vi "MotorControl.vi"() -> ()   [LabVIEW 2018]
panel:
  in  "stop":bool
  in  "Motor control":enum32{"Movement", "Setup", "Error"}(tab)
  in  "Single motion":bool=TRUE
  out "Step number":i32=1
  out "Motor Relative":dbl[](array[numeric])=[-100.0, -1.0, -1.0, -1.0]
  in  "Speed (mm/s)":dbl[](array[numeric])=[5.0, 5.0, 5.0, 10.0] format="%#_13g"
  in  "Distance  (mm)":dbl[](array[numeric])=[0.0, -100.0, 0.0, 0.0] format="%#_13g"
  in  "Send All":bool
  in  "Stop motion":bool
  out "Moving":bool
  out "Acquiring":bool
  in  "Go to zero":bool
  out "Motor Status":bool
  out "Number of steps":i32=1
  out "Time between steps":dbl format="%#_13g"
  out "run number":i32=37
  in  "Reset motor":bool
  in  "Inc run #":bool
  in  "Send":bool[](array[boolean])=[FALSE, FALSE, FALSE, FALSE]
  in  "Motor zero":dbl[](array[numeric])=[100.0, 1.0, 1.0, 1.0] format="%#_13g"
  out "Motor absolute":dbl[](array[numeric])
  in  "Motor Port":string="COM12 19200"
  in  "Time between steps ctrl":dbl=5.0 caption="Time Target (s)"
  in  "# steps ctrl":i32=3
  in  "Conversion (steps/mm)":dbl[](array[numeric])=[31496.063, 31496.063, 31496.063, 12500.0] format="%#_13g"
  in  "Reset distance after run":bool
  in  "auto inc run #":bool
  in  "Zero":bool[](array[boolean])=[FALSE, FALSE, FALSE, FALSE]
  out "error out":errorcluster={"status"=TRUE, "code"=-2147221164, "source"="Class not registered\r\n in MotorControl - Copy.vi"}
  out "Library Version":string
  out "Connect To:":string
  in  "Galil.IGalil":refnum<k7>
  # "spend time updating output cluster?"
  # "Motor A"
  # "Motor B"
  # "Motor C"
  # "Motor D"
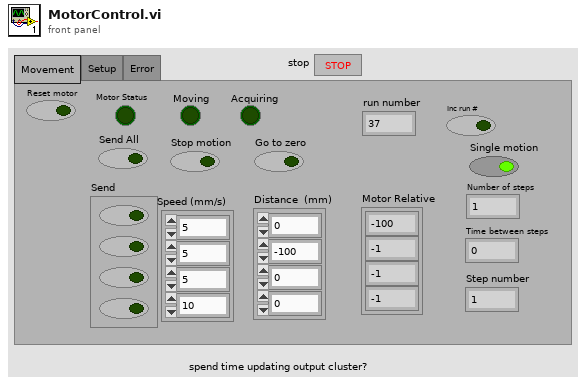
[diagram p1: front panel]
types:
  T1 = enum16{"open", "open or create", "create or replace", "create", "open (read-only)"}
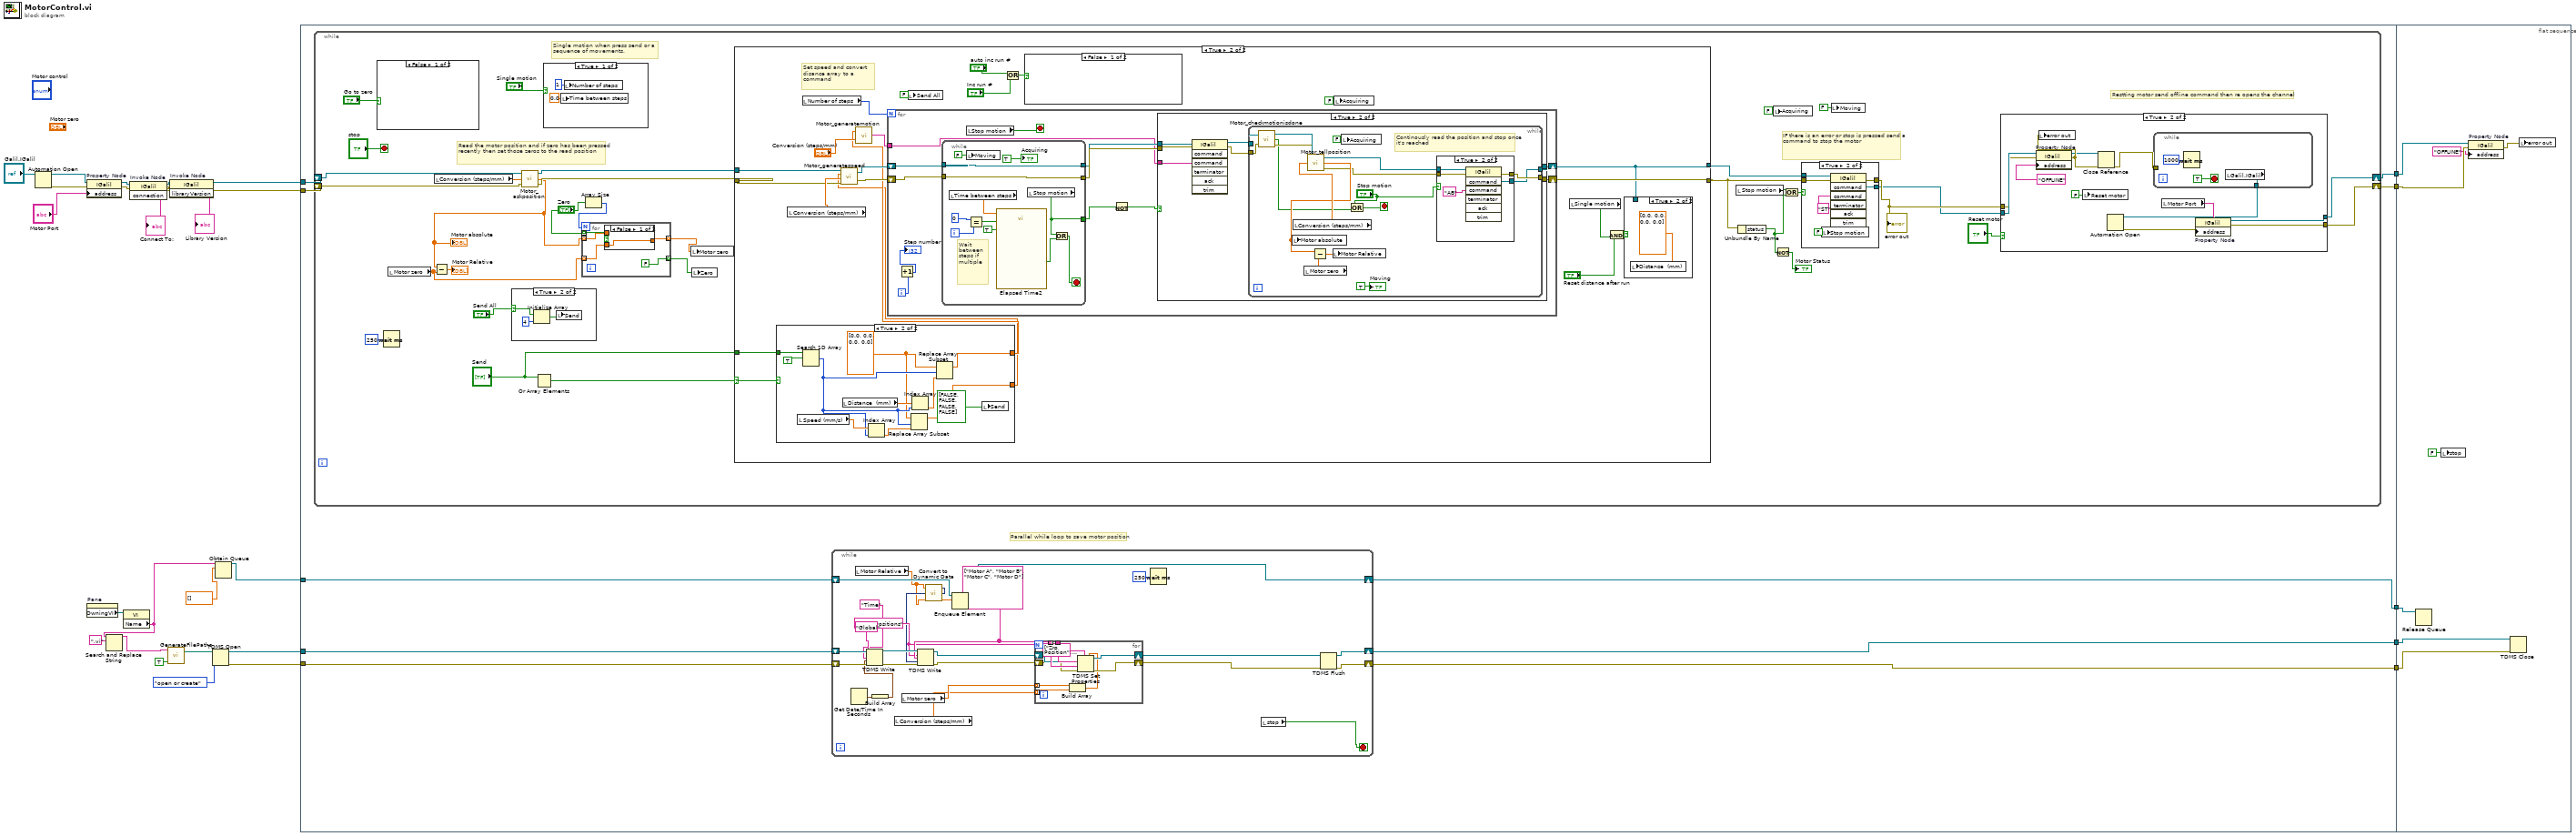
[diagram p0: block diagram]
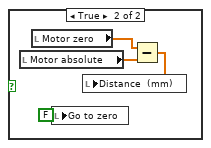
[diagram p5: hidden frame]
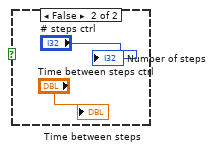
[diagram p7: hidden frame]
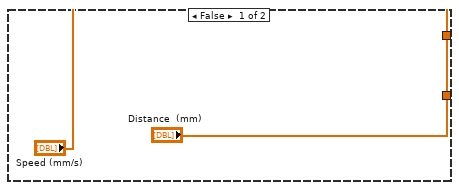
[diagram p9: hidden frame]
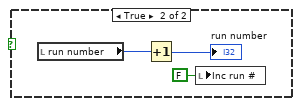
[diagram p10: hidden frame]
diagram:
  n1 = Automation Open(Automation Refnum="Galil.IGalil") -> (Automation Refnum=w22:refnum<k7>, error out=w26:errorcluster)  [unwired: 3 in]
  n2 = property on="Property Node" class="IGalil"(reference=w22, error in=w26, "address"="Motor Port") -> (reference out=w27:refnum<k7>, error out=w25:errorcluster)
  n3 = property on="Pane" class="Pane"() -> ("OwningVI"=w16:refnum<vi>)  [unwired: 2 in, 2 out]
  n4 = property class="VI"(reference=w16) -> ("Name"=w1:string)  [unwired: 1 in, 2 out]
  n5 = Search and Replace String(input string=w1, search string=".vi") -> (result string=w14:string)  [unwired: 6 in, 3 out]
  n6 = invoke on="Invoke Node" class="IGalil" method="connection"(reference=w27, error in=w25) -> (reference out=w21:refnum<k7>, error out=w20:errorcluster, "connection"=→"Connect To:":string)  [unwired: 1 in]
  n7 = call "GenerateFilePaths.vi"("Logfile? (F)"=TRUE ("Logfile?"), "Device Name"=w14) -> ("Path"=w12:path)  [unwired: 3 in]
  n8 = invoke on="Invoke Node" class="IGalil" method="libraryVersion"(reference=w21, error in=w20) -> (reference out=w18:refnum<k7>, error out=w17:errorcluster, "libraryVersion"=→"Library Version":string)  [unwired: 1 in]
  n9 = TDMS Open(10:T1."open or create" ("operation (0:open)"), 11:w12) -> (0:w9:errorcluster, 3:w10:refnum<k34>)  [unwired: 5 in]
  n10 = Obtain Queue(name (unnamed)=w1, element data type=dbl[] []) -> (queue out=w3:refnum<queue>)  [unwired: 3 in, 2 out]
  n11 = flat-sequence {
    tunnel: w18 -> [w38]
    tunnel: w17 -> [w37]
    tunnel: w10 -> [w34]
    tunnel: w9 -> [w33]
    tunnel: [w36] -> w8
    tunnel: [w35] -> w7
    tunnel: [w32] -> w6
    tunnel: [w31] -> w5
    tunnel: w3 -> [w29]
    tunnel: [w30] -> w2
    tunnel: w8 -> [w251]
    tunnel: w7 -> [w250]
    tunnel: w6 -> [w253]
    tunnel: w5 -> [w254]
    tunnel: w2 -> [w247]
    frame #0 {
      # "Parallel while loop to save motor position"
      n12 = while {
        shift-right: [w84] -> w36
        shift-left: w38 -> [w94]
        shift-right: [w83] -> w35
        shift-left: w37 -> [w93]
        stop <- "stop" stop-if-true
        # "Restting motor send offline command then re opens the channel"
        # "IF there is an error or stop is pressed send a command to stop the motor"
        # "Read the motor position and if zero has been pressed recently then set those zeros to the read position"
        # "Single motion when press send or a sequence of movements."
        n13 = case shown="False" "Go to zero" {
          frame False {
          }
          frame True {
            n14 = local read "Motor absolute"() -> (w134:dbl[])
            n15 = local read "Motor zero"() -> (w135:dbl[])
            n16 = local write "Go to zero"(FALSE ("Zero A")) -> ()
            n17 = Subtract(x=w135, y=w134) -> (x-y=w133:dbl[])
            n18 = local write "Distance  (mm)"(w133) -> ()
          }
        }
        n19 = Wait (ms)(milliseconds to wait=u32 250) -> ()  [unwired: 1 out]
        n20 = local read "Motor zero"() -> (w80:dbl[])
        n21 = local read "Conversion (steps/mm)"() -> (w90:dbl[])
        n22 = case shown="True" "Send All" {
          selector: "Send All" -> [_ w106]
          frame False {
          }
          frame True {
            n23 = Initialize Array(w106, 4 ("dimension size")) -> (w105:bool[])
            n24 = local write "Send"(w105) -> ()
          }
        }
        n25 = call "Motor_askposition.vi"("error in (no error)"=w93, "Conversion\n (steps/mm)"=w90, "reference"=w94) -> ("error out"=w91:errorcluster, "position out"=w73:dbl[], "reference out"=w92:refnum<k7>)
        "Motor absolute" <- w73
        n26 = Subtract(x=w73, y=w80) -> (x-y=→"Motor Relative":dbl[])
        n27 = Or Array Elements(Boolean array="Send") -> (logical OR=w77:bool)
        n28 = case shown="True" "Single motion" {
          frame True {
            n29 = local write "Time between steps"(0.0 ("Time between steps")) -> ()
            n30 = local write "Number of steps"(1 ("Number of steps")) -> ()
          }
          frame False {
            "Number of steps" <- "# steps ctrl"
            "Time between steps" <- "Time between steps ctrl"
          }
        }
        n31 = Array Size(array="Zero") -> (size(s)=w74:i32)
        n32 = for {
          N: w74 -> [_]
          tunnel: w73 -> [w112] mode=indexing
          tunnel: [FALSE ("Boolean")] -> w81 mode=indexing
          tunnel: "Zero" -> [w111] mode=indexing
          tunnel: [w110] -> w79 mode=indexing
          tunnel: w80 -> [w109] mode=indexing
          n33 = case shown="False" w111 {
            tunnel: w112 -> [_ w114]
            tunnel: [w113 w114] -> w110
            tunnel: w109 -> [w113 _]
            frame False {
            }
            frame True {
            }
          }
        }
        n34 = local write "Motor zero"(w79) -> ()
        n35 = local write "Zero"(w81) -> ()
        n36 = case shown="True" w77 {
          selector: w77 -> [_ w151]
          tunnel: w92 -> [w150 w164]
          tunnel: w91 -> [w149 w163]
          tunnel: [w150 w165] -> w98
          tunnel: [w149 w171] -> w95
          tunnel: "Send" -> [_ w154]
          frame False {
          }
          frame True {
            # "Set speed and convert disance array to a command"
            n37 = case shown="True" w151 {
              tunnel: w154 -> [_ w181]
              tunnel: ["Distance  (mm)" w180] -> w153
              tunnel: ["Speed (mm/s)" w176] -> w152
              frame False {
              }
              frame True {
                w175 = dbl[] [0.0, 0.0, 0.0, 0.0]
                n38 = local read "Speed (mm/s)"() -> (w178:dbl[])
                n39 = Search 1D Array(1D array=w181, element=TRUE) -> (index of element=w177:i32)  [unwired: 1 in]
                n40 = local read "Distance  (mm)"() -> (w183:dbl[])
                n41 = Index Array(array=w178, index=w177) -> (element=w179:dbl)
                n42 = Replace Array Subset(array=w175, new element=w179, index=w177) -> (w176:dbl[])
                n43 = Index Array(array=w183, index=w177) -> (element=w185:dbl)
                n44 = Replace Array Subset(array=w175, new element=w185, index=w177) -> (w180:dbl[])
                n45 = local write "Send"(bool[] [FALSE, FALSE, FALSE, FALSE]) -> ()
              }
            }
            n46 = local read "Conversion (steps/mm)"() -> (w166:dbl[])
            n47 = local read "Number of steps"() -> (w169:i32)
            n48 = call "Motor_generatespeed.vi"("error in (no error)"=w163, "Conversion\n (steps/mm)"=w166, "Speed (mm/s)"=w152, "reference"=w164) -> ("error out"=w161:errorcluster, "reference out"=w162:refnum<k7>)
            n49 = call "Motor_generatemotion.vi"("Conversion\n (steps/mm)"="Conversion (steps/mm)", "Distance  (mm)"=w153) -> ("Movement String"=w167:string)
            n50 = for {
              N: w169 -> [_]
              tunnel: w167 -> [w190]
              shift-right: [w196] -> w165
              shift-left: w162 -> [w198]
              shift-right: [w195] -> w171
              shift-left: w161 -> [w197]
              i -> [w200]
              stop <- w201 stop-if-true
              n51 = Increment(x=w200) -> (x+1=→"Step number":i32)
              n52 = while {
                tunnel: w198 -> [w245]
                tunnel: [w246] -> w192
                tunnel: w197 -> [w246]
                tunnel: [w245] -> w191
                tunnel: [w235] -> w193
                i -> [w241]
                stop <- w243 stop-if-true
                # "Wait between steps if multiple"
                n53 = local read "Time between steps"() -> (w237:dbl)
                n54 = local write "Moving"(FALSE ("Aquiring")) -> ()
                n55 = Equal?(x=0, y=w241) -> (x = y?=w239:bool)
                n56 = call "Elapsed Time2"("Time Target (s)"=w237, "Reset"=w239, "Auto Reset"=TRUE) -> ("Time has Elapsed"=w244:bool)  [unwired: 9 in, 7 out]
                n57 = local read "Stop motion"() -> (w235:bool)
                n58 = Or(x=w235, y=w244) -> (x .or. y?=w243:bool)
                "Acquiring" <- TRUE
              }
              n59 = local read "Stop motion"() -> (w201:bool)
              n60 = Not(x=w193) -> (.not. x?=w194:bool)
              n61 = case shown="True" w194 {
                tunnel: w191 -> [w203 w208]
                tunnel: w192 -> [w202 w205]
                tunnel: [w203 w210] -> w196
                tunnel: [w202 w209] -> w195
                tunnel: w190 -> [_ w204]
                frame False {
                }
                frame True {
                  n62 = invoke class="IGalil" method="command"(reference=w208, error in=w205, "command"=w204) -> (reference out=w207:refnum<k7>, error out=w206:errorcluster)  [unwired: 4 in, 5 out]
                  n63 = while {
                    tunnel: w207 -> [w220]
                    tunnel: [w213] -> w210
                    tunnel: [w214] -> w209
                    tunnel: w206 -> [w211]
                    stop <- w226 stop-if-true
                    # "Continously read the position and stop once it's reached"
                    n64 = call "Motor_checkmotionisdone.vi"("reference"=w220, "error in (no error)"=w211) -> ("reference out"=w219:refnum<k7>, "Motion is done"=w217:bool, "error out"=w218:errorcluster)
                    n65 = local read "Conversion (steps/mm)"() -> (w222:dbl[])
                    n66 = local read "Motor zero"() -> (w225:dbl[])
                    n67 = call "Motor_tellposition.vi"("error in (no error)"=w218, "Conversion\n (steps/mm)"=w222, "reference"=w219) -> ("error out"=w215:errorcluster, "Position out"=w221:dbl[], "reference out"=w216:refnum<k7>)
                    n68 = local write "Motor absolute"(w221) -> ()
                    n69 = Subtract(x=w221, y=w225) -> (x-y=w224:dbl[])
                    n70 = local write "Motor Relative"(w224) -> ()
                    n71 = local write "Acquiring"(FALSE ("Aquiring")) -> ()
                    n72 = Or(x="Stop motion", y=w217) -> (x .or. y?=w226:bool)
                    n73 = case shown="True" "Stop motion" {
                      tunnel: w216 -> [w229 w233]
                      tunnel: w215 -> [w228 w232]
                      tunnel: [w229 w231] -> w213
                      tunnel: [w228 w230] -> w214
                      frame False {
                      }
                      frame True {
                        n74 = invoke class="IGalil" method="command"(reference=w233, error in=w232, "command"="AB") -> (reference out=w231:refnum<k7>, error out=w230:errorcluster)  [unwired: 4 in, 5 out]
                      }
                    }
                    "Moving" <- TRUE
                  }
                }
              }
            }
            n75 = local write "Send All"(FALSE ("Send")) -> ()
            n76 = Or(x="auto inc run #", y="Inc run #") -> (x .or. y?=w157:bool)
            n77 = case shown="False" w157 {
              frame False {
              }
              frame True {
                n78 = local read "run number"() -> (w187:i32)
                n79 = Increment(x=w187) -> (x+1=→"run number":i32)
                n80 = local write "Inc run #"(FALSE ("Inc run #")) -> ()
              }
            }
            n81 = local write "Acquiring"(FALSE ("Aquiring")) -> ()
            n82 = local read "Single motion"() -> (w159:bool)
            n83 = And(x="Reset distance after run", y=w159) -> (x .and. y?=w160:bool)
            n84 = case shown="True" w160 {
              tunnel: w165 -> [_ _]
              frame False {
              }
              frame True {
                n85 = local write "Distance  (mm)"(dbl[] [0.0, 0.0, 0.0, 0.0] ("Distance  (mm)")) -> ()
              }
            }
          }
        }
        n86 = local read "Stop motion"() -> (w96:bool)
        n87 = Unbundle By Name(w95) -> ("status"=w88:bool)
        n88 = local write "Acquiring"(FALSE ("Aquiring")) -> ()
        n89 = Not(x=w88) -> (.not. x?=→"Motor Status":bool)
        n90 = Or(x=w96, y=w88) -> (x .or. y?=w97:bool)
        n91 = case shown="True" w97 {
          tunnel: w98 -> [w138 w143]
          tunnel: w95 -> [w137 w142]
          tunnel: [w138 w141] -> w85
          tunnel: [w137 w140] -> w86
          frame False {
          }
          frame True {
            n92 = local write "Stop motion"(FALSE ("Stop motion")) -> ()
            n93 = invoke class="IGalil" method="command"(reference=w143, error in=w142, "command"="ST") -> (reference out=w141:refnum<k7>, error out=w140:errorcluster)  [unwired: 4 in, 5 out]
          }
        }
        "error out" <- w86
        n94 = local write "Moving"(FALSE ("Waiting")) -> ()
        n95 = case shown="True" "Reset motor" {
          tunnel: w85 -> [w115 w118]
          tunnel: w86 -> [w116 w117]
          tunnel: [w115 w128] -> w84
          tunnel: [w116 w129] -> w83
          frame False {
          }
          frame True {
            n96 = property on="Property Node" class="IGalil"(reference=w118, error in=w117, "address"="OFFLINE") -> (reference out=w121:refnum<k7>, error out=w122:errorcluster)
            n97 = local write "error out"(w122) -> ()
            n98 = local write "Reset motor"(FALSE ("Reset motor")) -> ()
            n99 = Close Reference(reference=w121, error in (no error)=w122) -> (error out=w119:errorcluster)
            n100 = while {
              tunnel: [w130] -> w126
              tunnel: w119 -> [_]
              stop <- TRUE stop-if-true
              n101 = Wait (ms)(milliseconds to wait=u32 1000) -> ()  [unwired: 1 out]
              n102 = local read "Galil.IGalil"() -> (w130:refnum<k7>)
            }
            n103 = Automation Open(Automation Refnum=w126) -> (Automation Refnum=w125:refnum<k7>, error out=w124:errorcluster)  [unwired: 3 in]
            n104 = local read "Motor Port"() -> (w127:string)
            n105 = property on="Property Node" class="IGalil"(reference=w125, error in=w124, "address"=w127) -> (reference out=w128:refnum<k7>, error out=w129:errorcluster)
          }
        }
      }
      n106 = while {
        shift-right: [w47] -> w32
        shift-left: w34 -> [w62]
        shift-right: [w48] -> w31
        shift-left: w33 -> [w61]
        shift-right: [w40] -> w30
        shift-left: w29 -> [w41]
        stop <- w46 stop-if-true
        w54 = string[] ["Motor A", "Motor B", "Motor C", "Motor D"]
        w53 = "Motor Positions" ("group name in (Untitled)")
        n107 = Get Date/Time In Seconds() -> (seconds since 1Jan1904=w58:timestamp)
        n108 = local read "Motor Relative"() -> (w39:dbl[])
        n109 = Build Array(w58) -> (w57:timestamp[])
        n110 = TDMS Write(0:w62, 5:"Global" ("group name in (Untitled)"), 7:"Time" ("group name in (Untitled)"), 9:w57, 11:w61) -> (4:w56:refnum<k34>, 15:w55:errorcluster)  [unwired: 1 in, 2 out]
        n111 = local read "Conversion (steps/mm)"() -> (w42:dbl[])
        n112 = local read "Motor zero"() -> (w43:dbl[])
        n113 = call "Convert to Dynamic Data"("Array"=w39) -> ("Dynamic Data Type"=w44:dynamicdata)  [unwired: 3 in]
        n114 = TDMS Write(0:w56, 5:w53, 7:w54, 9:w44, 11:w55) -> (4:w52:refnum<k34>, 15:w51:errorcluster)  [unwired: 1 in, 2 out]
        n115 = Enqueue Element(queue=w41, element=w39) -> (queue out=w40:refnum<queue>)  [unwired: 2 in, 2 out]
        n116 = for {
          tunnel: w54 -> [w72] mode=indexing
          tunnel: w53 -> [w71]
          shift-right: [w66] -> w49
          shift-left: w51 -> [w68]
          shift-right: [w67] -> w50
          shift-left: w52 -> [w69]
          tunnel: w43 -> [w65] mode=indexing
          tunnel: w42 -> [w64] mode=indexing
          n117 = Build Array(w65, w64) -> (w63:dbl[])
          n118 = TDMS Set Properties(5:w63, 7:string[] ["Zro Position", "Conversion (st/mm)"] ("property names"), 8:w68, 9:w72, 10:w71, 11:w69) -> (0:w66:errorcluster, 3:w67:refnum<k34>)  [unwired: 2 out]
        }
        n119 = Wait (ms)(milliseconds to wait=u32 250) -> ()  [unwired: 1 out]
        n120 = local read "stop"() -> (w46:bool)
        n121 = TDMS Flush(4:w49, 7:w50) -> (0:w48:errorcluster, 3:w47:refnum<k34>)
      }
    }
    frame #1 {
      n122 = Release Queue(queue=w247) -> ()  [unwired: 2 in, 3 out]
      n123 = local write "stop"(FALSE ("stop")) -> ()
      n124 = property on="Property Node" class="IGalil"(reference=w251, error in=w250, "address"="OFFLINE") -> (error out=w252:errorcluster)  [unwired: 1 out]
      n125 = TDMS Close(8:w254, 11:w253) -> ()  [unwired: 2 out]
      n126 = local write "error out"(w252) -> ()
    }
  }
